vi "Prepare_plots_SubVI_v1.vi"(6 "Signal in X or Y (?)":bool, 8 "Y rot avg in":dbl[](array[numeric]), 9 "X rot avg in":dbl[](array[numeric]), 10 "Cutted Data 3":T1, 11 "Cutted Data 0":T1) -> (0 "Y rot avg out":dbl[](array[numeric]), 1 "X rot avg out":dbl[](array[numeric]), 2 "Monitor":cluster{"Time":dbl[], dbl[]}, 3 "RF out":cluster{"Time":dbl[], "Y":dbl[]}[](array[cluster]), 4 "Rotation spectrum":waveform(dbl)[](array[waveform]), 5 "Rotation":cluster{"Time":dbl[], dbl[]}[](array[cluster]), 7 "Polarimeter":dbl format="%0.2f")   [LabVIEW 2021]
uses:
  Ver_2/Cutted_Data_v2.ctl
  <vilib>/Analysis/baseanly.llb/Mean (DBL).vi
  <vilib>/Analysis/NI_AALPro.lvlib
  <vilib>/Analysis/NI_AALBase.lvlib
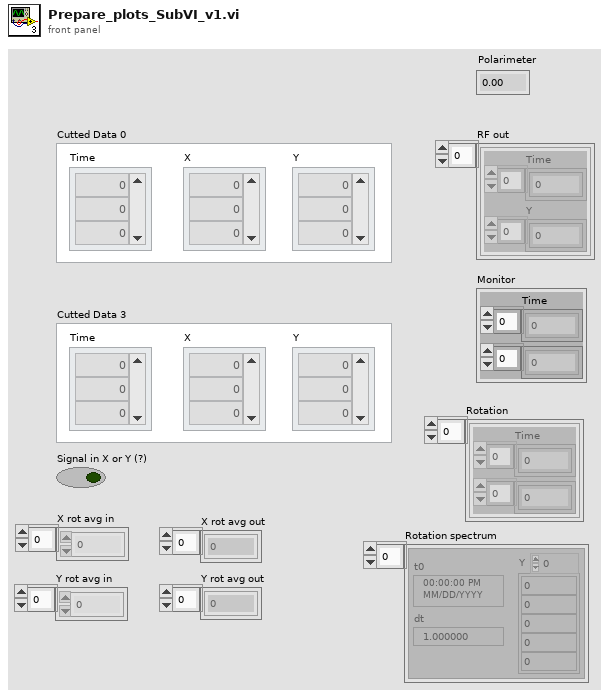
[diagram p1: front panel]
types:
  T1 = typedef "Cutted_Data_v2.ctl" = cluster{"X":dbl[], "Y":dbl[], "Time":dbl[]}
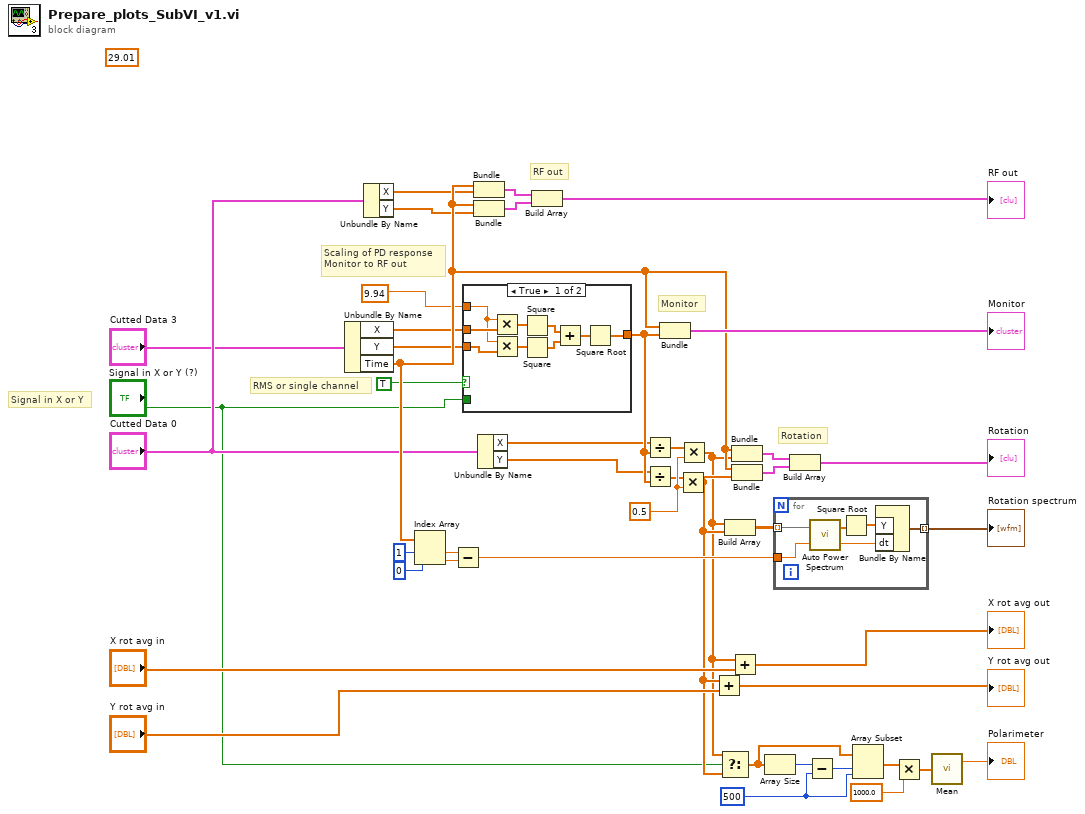
[diagram p0: block diagram]
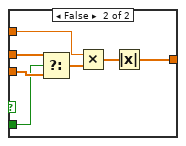
[diagram p2: hidden frame]
diagram:
  (unwired) 29.01
  w7 = 500
  w31 = 0.5
  # "Rotation"
  # "Monitor"
  # "RF out"
  # "RMS or single channel"
  # "Signal in X or Y"
  # "Scaling of PD response\nMonitor to RF out"
  n1 = Unbundle By Name("Cutted Data 3") -> ("X"=w18:dbl[], "Y"=w17:dbl[], "Time"=w34:dbl[])
  n2 = Unbundle By Name("Cutted Data 0") -> ("X"=w24:dbl[], "Y"=w25:dbl[])
  n3 = Index Array(array=w34, index #1=1 ("index"), index #2=0 ("index")) -> (element #1=w14:dbl, element #2=w13:dbl)
  n4 = Subtract(x=w14, y=w13) -> (x-y=w38:dbl)
  n5 = case shown="True" TRUE {
    tunnel: w17 -> [w48 w58]
    tunnel: w18 -> [w47 w57]
    tunnel: 9.94 -> [w46 w56]
    tunnel: [w45 w55] -> w28
    tunnel: "Signal in X or Y (?)" -> [_ w54]
    frame True {
      n6 = Multiply(x=w46, y=w47) -> (x*y=w50:dbl[])
      n7 = Multiply(x=w46, y=w48) -> (x*y=w49:dbl[])
      n8 = Square(x=w50) -> (x^2=w51:dbl[])
      n9 = Square(x=w49) -> (x^2=w52:dbl[])
      n10 = Add(x=w51, y=w52) -> (x+y=w53:dbl[])
      n11 = Square Root(x=w53) -> (sqrt(x)=w45:dbl[])
    }
    frame False {
      n12 = Select(t=w57, s=w54, f=w58) -> (s? t:f=w59:dbl[])
      n13 = Multiply(x=w56, y=w59) -> (x*y=w60:dbl[])
      n14 = Absolute Value(x=w60) -> (abs(x)=w55:dbl[])
    }
  }
  n15 = Bundle("Time"=w34, "X"=w24) -> (w21:cluster{"Time":dbl[], "X":dbl[]})  [unwired: 1 in]
  n16 = Bundle("Time"=w34, "Y"=w25) -> (w22:cluster{"Time":dbl[], "Y":dbl[]})  [unwired: 1 in]
  n17 = Unbundle By Name("Cutted Data 0") -> ("X"=w26:dbl[], "Y"=w27:dbl[])
  n18 = Build Array(w21, w22) -> (→"RF out":cluster{"Time":dbl[], "Y":dbl[]}[])
  n19 = Divide(x=w26, y=w28) -> (x/y=w30:dbl[])
  n20 = Divide(x=w27, y=w28) -> (x/y=w29:dbl[])
  n21 = Bundle("Time"=w34, w28) -> (→"Monitor":cluster{"Time":dbl[], dbl[]})  [unwired: 1 in]
  n22 = Multiply(x=w29, y=w31) -> (x*y=w12:dbl[])
  n23 = Multiply(x=w30, y=w31) -> (x*y=w11:dbl[])
  n24 = Add(x=w12, y="Y rot avg in") -> (x+y=→"Y rot avg out":dbl[])
  n25 = Select(t=w11, s="Signal in X or Y (?)", f=w12) -> (s? t:f=w6:dbl[])
  n26 = Build Array(w11, w12) -> (w39:dbl[][])
  n27 = Add(x=w11, y="X rot avg in") -> (x+y=→"X rot avg out":dbl[])
  n28 = Bundle("Time"=w34, w11) -> (w33:cluster{"Time":dbl[], dbl[]})  [unwired: 1 in]
  n29 = Bundle("Time"=w34, w12) -> (w32:cluster{"Time":dbl[], dbl[]})  [unwired: 1 in]
  n30 = Array Size(array=w6) -> (size(s)=w9:i32)
  n31 = for {
    tunnel: w39 -> [w66] mode=indexing
    tunnel: [w64] -> w40 mode=indexing
    tunnel: w38 -> [w61]
    n32 = call <vilib>:"Auto Power Spectrum.vi"("dt"=w61, "Signal (V)"=w66) -> ("df"=w65:dbl, "Power Spectrum (V^2 rms)"=w63:dbl[])
    n33 = Square Root(x=w63) -> (sqrt(x)=w62:dbl[])
    n34 = Bundle By Name("Y"=w62, "dt"=w65) -> (w64:waveform(dbl))  [unwired: 1 in]
  }
  "Rotation spectrum" <- w40
  n35 = Build Array(w33, w32) -> (→"Rotation":cluster{"Time":dbl[], dbl[]}[])
  n36 = Subtract(x=w9, y=w7) -> (x-y=w8:i32)
  n37 = Array Subset(array=w6, index=w8, length=w7) -> (w5:dbl[])
  n38 = Multiply(x=w5, y=1000.0) -> (x*y=w3:dbl[])
  n39 = call-poly <vilib>:"Mean.vi"("X"=w3) -> ("mean"=→"Polarimeter":dbl)  [unwired: 1 out]
